vi "Keithley 2600 Series Current Sweep.vi"() -> ()   [LabVIEW 2017]
doc: "This example shows how to create, run a script and query the script output data."
uses:
  <vilib>/Utility/file.llb/Write Delimited Spreadsheet (DBL).vi
  <instrlib>/Keithley 2600 Series/Keithley 2600 Series.lvlib
panel:
  out "output array":string[][](array[string])
  out "Graph 2":cluster{"Y":dbl[], "Y":dbl[]}[](graph)
  out "Working Folder":path
  in  "Folder Name":string="Raw Measurement"
  in  "Cluster":T1={"Start Voltage(V)"=0.0, "Stop Voltage(V)"=0.0, "Number of Points"=10.0, "Settling Time(s)"=0.1, "Current Limit(A)"=0.1} {"Current Limit(A)" min=0.1 max=1.5; "Settling Time(s)" min=0.1 max=60.0; "Number of Points" min=10.0 max=10000.0 step=1.0; "Stop Voltage(V)" min=0.0 max=200.0; "Start Voltage(V)" min=0.0 max=200.0}
  in  "VISA resource name":refnum<visa-resource-name>
  # "Sweep Setting (Channel A)"
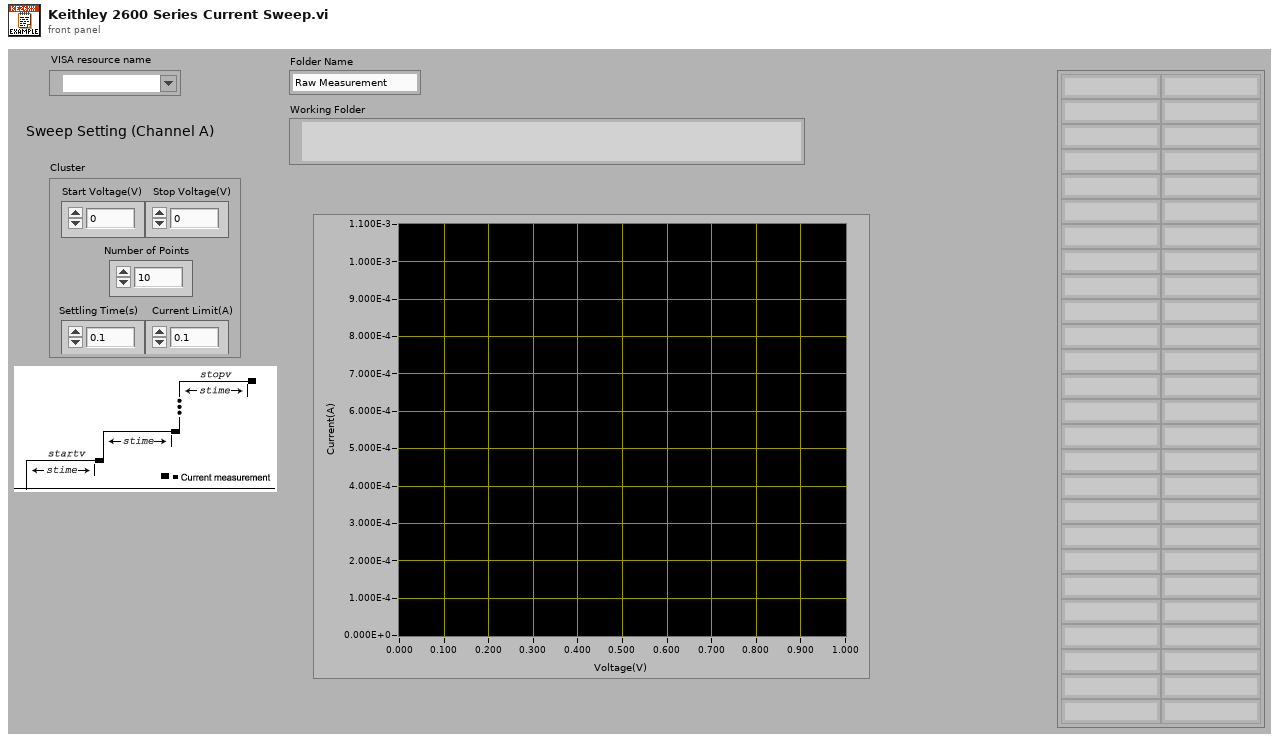
[diagram p1: front panel]
types:
  T1 = cluster{"Start Voltage(V)":dbl, "Stop Voltage(V)":dbl, "Number of Points":dbl, "Settling Time(s)":dbl, "Current Limit(A)":dbl}
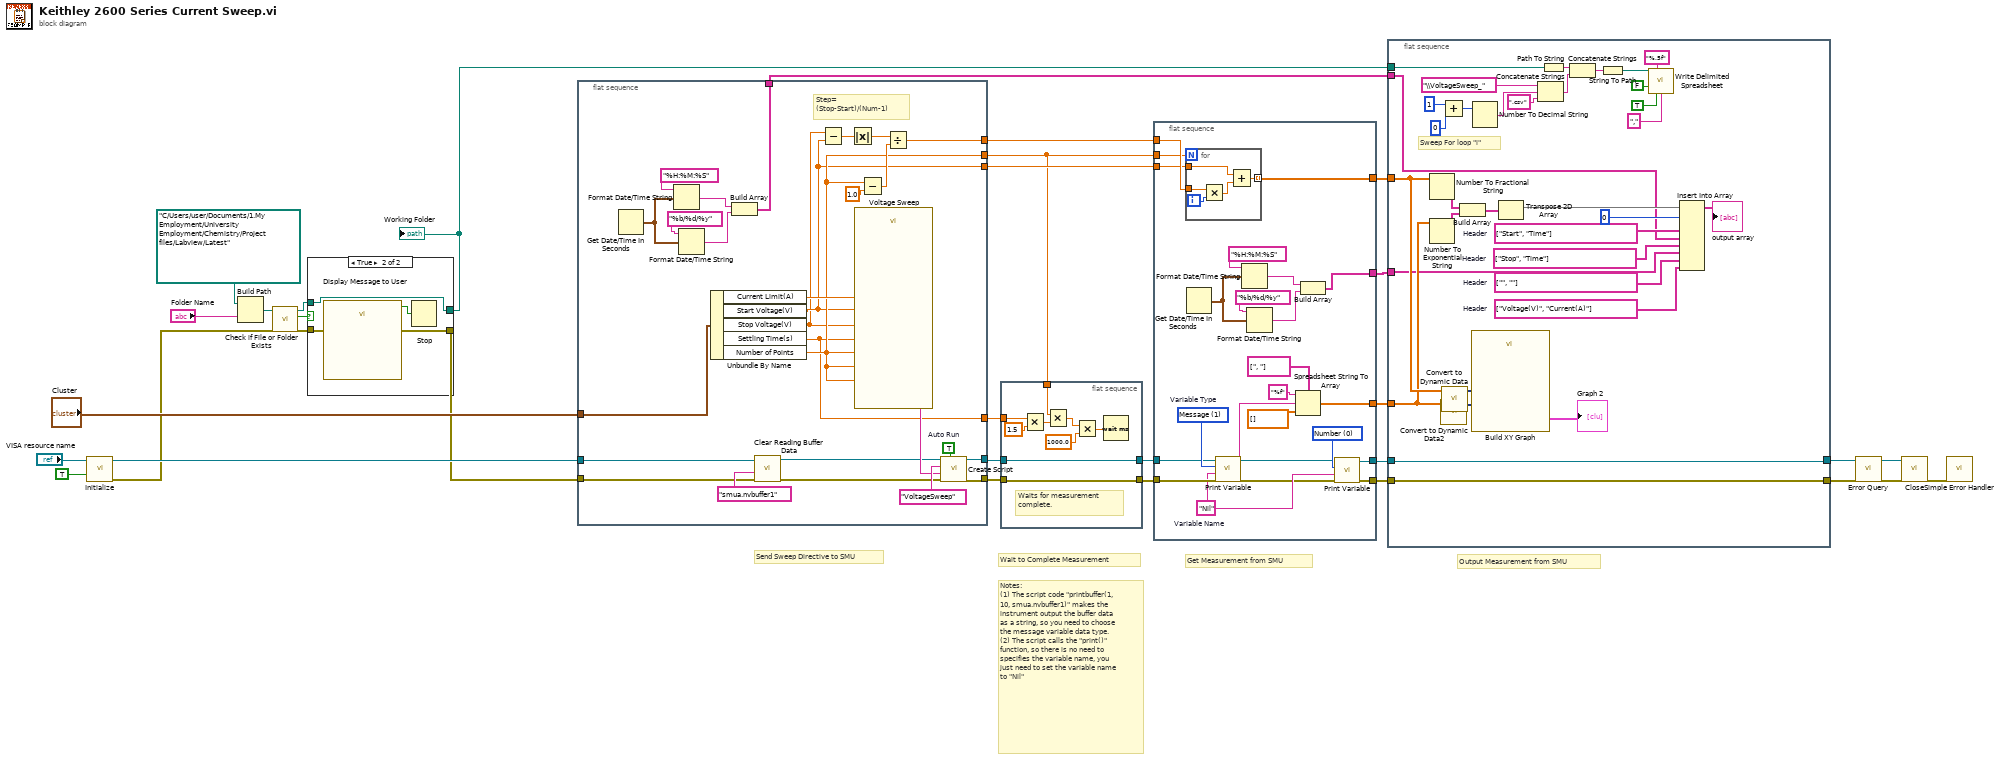
[diagram p0: block diagram]
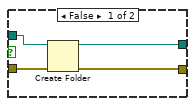
[diagram p2: hidden frame]
diagram:
  # "Send Sweep Directive to SMU"
  # "Wait to Complete Measurement"
  # "Output Measurement from SMU"
  # "Get Measurement from SMU"
  # "Notes: \n(1) The script code \"printbuffer(1, 10, smua.nvbuffer1)\" makes the instrument output the buffer data as a string, so you need to choose the message variable data type.\n(2) The script calls the \"print()\" function, so there is no need to specifies the variable name, you just need to set the variable name to \"Nil\""
  n1 = call <instrlib>:"Initialize.vi"("Reset (True)"=TRUE, "VISA resource name"="VISA resource name") -> ("error out"=w15:errorcluster, "VISA resource name out"=w24:refnum<visa-resource-name>)  [unwired: 8 in]
  n2 = Build Path(base path=path "C:/Users/user/Documents/1.My Employment/University Employment/Chemistry/Project files/Labview/Latest" ("Working Directory"), name or relative path="Folder Name") -> (appended path=w19:path)
  n3 = call <vilib>:"Check if File or Folder Exists.vi"("error in (no error)"=w15, "path"=w19) -> ("error out"=w16:errorcluster, "file or folder exists?"=w18:bool, "dup path"=w17:path)  [unwired: 7 in]
  n4 = case shown="True" w18 {
    tunnel: [w35 w38] -> w13
    tunnel: w17 -> [w36 w38]
    tunnel: w16 -> [w34 w40]
    tunnel: [w33 w37] -> w14
    frame False {
      n5 = Create Folder(path (use dialog)=w36, error in=w34) -> (created path=w35:path, error out=w33:errorcluster)  [unwired: 1 in, 1 out]
    }
    frame True {
      n6 = call "Display Message to User"("error in (no error)"=w40) -> ("error out"=w37:errorcluster, "OK"=w39:bool)  [unwired: 9 in]
      n7 = Stop(stop? (T)=w39) -> ()
    }
  }
  "Working Folder" <- w13
  n8 = flat-sequence {
    tunnel: "Cluster" -> [w66]
    tunnel: [w52] -> w6
    tunnel: [w53] -> w5
    tunnel: w24 -> [w65]
    tunnel: [w59] -> w23
    tunnel: w14 -> [w58]
    tunnel: [w43] -> w11
    tunnel: [w57] -> w4
    tunnel: [w41] -> w3
    tunnel: [w44] -> w2
    frame #0 {
      w55 = TRUE  # Auto Run
      # "Step=\n(Stop-Start)/(Num-1)"
      n9 = Get Date/Time In Seconds() -> (seconds since 1Jan1904=w45:timestamp)
      n10 = Format Date/Time String(time format string (%c)="%H:%M:%S", seconds (now)=w45) -> (date/time string=w48:string)  [unwired: 1 out]
      n11 = Format Date/Time String(time format string (%c)="%b/%d/%y", seconds (now)=w45) -> (date/time string=w46:string)  [unwired: 1 out]
      n12 = Unbundle By Name(w66) -> ("Current Limit(A)"=w67:dbl, "Start Voltage(V)"=w43:dbl, "Stop Voltage(V)"=w42:dbl, "Settling Time(s)"=w41:dbl, "Number of Points"=w57:dbl)
      n13 = Build Array(w48, w46) -> (w44:string[])
      n14 = call <instrlib>:"Clear Reading Buffer Data.vi"("error in (no error)"=w58, "Reading Buffer (smua.nvbuffer1)"="smua.nvbuffer1", "VISA resource name"=w65) -> ("error out"=w50:errorcluster, "VISA resource name out"=w51:refnum<visa-resource-name>)  [unwired: 7 in]
      n15 = Subtract(x=w42, y=w43) -> (x-y=w62:dbl)
      n16 = Absolute Value(x=w62) -> (abs(x)=w61:dbl)
      n17 = call "Voltage Sweep"("StopV"=w42, "LevelNumber1"=w57, "CurrentLimit"=w67, "SettlingTime"=w41, "StartV"=w43, "LevelNumber0"=w57, "LevelNumber2"=w57) -> ("Result"=w54:string)  [unwired: 7 in, 1 out]
      n18 = Subtract(x=w57, y=1.0) -> (x-y=w63:dbl)
      n19 = Divide(x=w61, y=w63) -> (x/y=w59:dbl)
      n20 = call <instrlib>:"Create Script.vi"("Auto Run (F: Disable)"=w55, "error in (no error)"=w50, "Source Code"=w54, "Script Variable"="VoltageSweep", "VISA resource name"=w51) -> ("error out"=w53:errorcluster, "VISA resource name out"=w52:refnum<visa-resource-name>)  [unwired: 5 in]
    }
  }
  n21 = flat-sequence {
    tunnel: w6 -> [w75]
    tunnel: w5 -> [w76]
    tunnel: [w76] -> w30
    tunnel: [w75] -> w31
    tunnel: w4 -> [w74]
    tunnel: w3 -> [w73]
    frame #0 {
      # "Waits for measurement complete."
      n22 = Multiply(x=w73, y=1.5) -> (x*y=w71:dbl)
      n23 = Multiply(x=w74, y=w71) -> (x*y=w70:dbl)
      n24 = Multiply(x=w70, y=1000.0) -> (x*y=w69:dbl)
      n25 = Wait (ms)(milliseconds to wait=w69) -> ()  [unwired: 1 out]
    }
  }
  n26 = flat-sequence {
    tunnel: w31 -> [w99]
    tunnel: w30 -> [w98]
    tunnel: w23 -> [w93]
    tunnel: [w92] -> w22
    tunnel: [w90] -> w12
    tunnel: w11 -> [w89]
    tunnel: w4 -> [w88]
    tunnel: [w84] -> w10
    tunnel: [w83] -> w7
    tunnel: [w77] -> w1
    frame #0 {
      w86 = 0 items=["Number", "Message"] ("Variable Type (0: Number)")
      w100 = 1 items=["Number", "Message"]  # Variable Type
      w91 = "Nil"  # Variable Name
      n27 = for {
        N: w88 -> [_]
        tunnel: w93 -> [w104]
        tunnel: w89 -> [w102]
        tunnel: [w101] -> w90 mode=indexing
        i -> [w105]
        n28 = Multiply(x=w104, y=w105) -> (x*y=w103:dbl)
        n29 = Add(x=w102, y=w103) -> (x+y=w101:dbl)
      }
      n30 = Get Date/Time In Seconds() -> (seconds since 1Jan1904=w78:timestamp)
      n31 = call <instrlib>:"Print Variable.vi"("error in (no error)"=w98, "Variable Name"=w91, "Variable Type (0: Number)"=w100, "VISA resource name"=w99) -> ("error out"=w87:errorcluster, "Message"=w97:string, "VISA resource name out"=w85:refnum<visa-resource-name>)  [unwired: 4 in, 1 out]
      n32 = Format Date/Time String(time format string (%c)="%H:%M:%S", seconds (now)=w78) -> (date/time string=w81:string)  [unwired: 1 out]
      n33 = Format Date/Time String(time format string (%c)="%b/%d/%y", seconds (now)=w78) -> (date/time string=w79:string)  [unwired: 1 out]
      n34 = Spreadsheet String To Array(delimiter (Tab)=string[] [", "], format string="%f", spreadsheet string=w97, array type (2D Dbl)=dbl[] []) -> (array=w92:dbl[])
      n35 = Build Array(w81, w79) -> (w77:string[])
      n36 = call <instrlib>:"Print Variable.vi"("error in (no error)"=w87, "Variable Name"=w91, "Variable Type (0: Number)"=w86, "VISA resource name"=w85) -> ("error out"=w84:errorcluster, "VISA resource name out"=w83:refnum<visa-resource-name>)  [unwired: 4 in, 2 out]
    }
  }
  n37 = flat-sequence {
    tunnel: w22 -> [w116]
    tunnel: w13 -> [w121]
    tunnel: w12 -> [w117]
    tunnel: w10 -> [w123]
    tunnel: [w123] -> w9
    tunnel: [w122] -> w8
    tunnel: w7 -> [w122]
    tunnel: w2 -> [w110]
    tunnel: w1 -> [w109]
    frame #0 {
      w106 = string[] ["Voltage(V)", "Current(A)"]  # Header
      w107 = string[] ["", ""]  # Header
      w108 = string[] ["Stop", "Time"]  # Header
      w112 = string[] ["Start", "Time"]  # Header
      # "Sweep For loop \"i\""
      n38 = Number To Fractional String(number=w117) -> (F-format string=w119:string[])  [unwired: 3 in]
      n39 = Number To Exponential String(number=w116) -> (E-format string=w118:string[])  [unwired: 3 in]
      n40 = Add(x=1, y=0) -> (x+y=w125:i32)
      n41 = call "Convert to Dynamic Data2"("Array"=w116) -> ("Dynamic Data Type"=w138:dynamicdata)  [unwired: 3 in]
      n42 = call "Convert to Dynamic Data"("Array"=w117) -> ("Dynamic Data Type"=w139:dynamicdata)  [unwired: 3 in]
      n43 = Build Array(w119, w118) -> (w120:string[][])
      n44 = call "Build XY Graph"("Y Input"=w138, "X Input"=w139) -> ("XY Graph"=→"Graph 2":cluster{"X":dbl[], "Y":dbl[]}[])  [unwired: 8 in, 1 out]
      n45 = Number To Decimal String(number=w125) -> (decimal integer string=w126:string)  [unwired: 1 in]
      n46 = Transpose 2D Array(2D array=w120) -> (transposed array=w114:string[][])
      n47 = Concatenate Strings("\\VoltageSweep_" ("string"), w126, ".csv" ("string")) -> (w130:string)
      n48 = Path To String(path=w121) -> (string=w136:string)
      n49 = Concatenate Strings(w136, w130) -> (w135:string)
      n50 = String To Path(string=w135) -> (path=w134:path)
      n51 = call-poly <vilib>:"Write Delimited Spreadsheet.vi"("file path (dialog if empty)"=w134, "format (%.3f)"="%.5f", "append to file? (new file:F)"=FALSE, "transpose? (no:F)"=TRUE, "delimiter (\\t)"="," ("delimiter (\\t)")) -> ()  [unwired: 9 in, 2 out]
      n52 = Insert Into Array(array=w114, index (row)=0, new element #1=w112, new element #2=w110, new element #3=w108, new element #4=w109, new element #5=w107, new element #6=w106) -> (→"output array":string[][])  [unwired: 1 in]
    }
  }
  n53 = call <instrlib>:"Error Query.vi"("error in (no error)"=w9, "VISA resource name"=w8) -> ("error out"=w28:errorcluster, "VISA resource name out"=w29:refnum<visa-resource-name>)  [unwired: 6 in, 2 out]
  n54 = call <instrlib>:"Close.vi"("error in (no error)"=w28, "VISA resource name"=w29) -> ("error out"=w32:errorcluster)  [unwired: 9 in]
  n55 = call <vilib>:"Simple Error Handler.vi"("error in (no error)"=w32) -> ()  [unwired: 4 in, 5 out]
